vi "Calculate Grid Size.vi"(0 "Rope Data":T1) -> (1 "Rows":i32, 2 "Columns":i32, 3 "Offset":cdb)   [LabVIEW 2020, in "AoC 2022.lvlib"]
uses:
  AoC 2022.lvlib
  Rope Data.ctl
  Positions.ctl
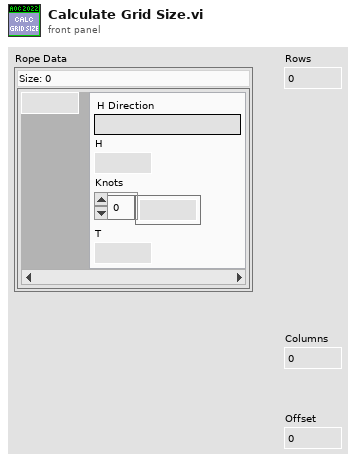
[diagram p1: front panel]
types:
  T1 = typedef "AoC 2022.lvlib/Rope Data.ctl" = map{i32, T2}
  T2 = typedef "AoC 2022.lvlib/Positions.ctl" = cluster{"H Direction":string, "H":cdb, "Knots":cdb[], "T":cdb}
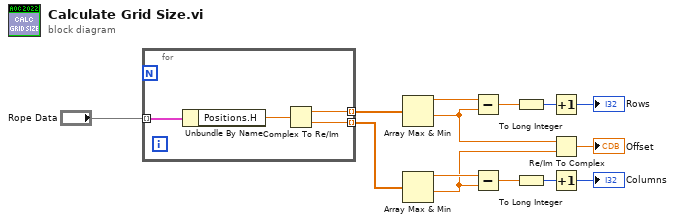
[diagram p0: block diagram]
diagram:
  n1 = for {
    tunnel: "Rope Data" -> [w18] mode=indexing
    tunnel: [w16] -> w11 mode=indexing
    tunnel: [w15] -> w10 mode=indexing
    n2 = Unbundle By Name(w18) -> ("Positions.H"=w17:cdb)
    n3 = Complex To Re/Im(x + iy=w17) -> (x=w16:dbl, y=w15:dbl)
  }
  n4 = Array Max & Min(array=w11) -> (max value=w9:dbl, min value=w3:dbl)  [unwired: 2 out]
  n5 = Array Max & Min(array=w10) -> (max value=w8:dbl, min value=w2:dbl)  [unwired: 2 out]
  n6 = Subtract(x=w9, y=w3) -> (x-y=w7:dbl)
  n7 = Subtract(x=w8, y=w2) -> (x-y=w6:dbl)
  n8 = To Long Integer(number=w7) -> (32bit integer=w13:i32)
  n9 = To Long Integer(number=w6) -> (32bit integer=w12:i32)
  n10 = Increment(x=w13) -> (x+1=→"Rows":i32)
  n11 = Re/Im To Complex(1:w2, 2:w3) -> (0:→"Offset":cdb)
  n12 = Increment(x=w12) -> (x+1=→"Columns":i32)
